vi "Configure Thermistor [THM].vi"(8 "error in (no error)":errorcluster, 10 "resistance (0.0 ohms)":dbl format="%^.2e", 11 "CS++DMM in":refnum<class "CS++DMM.lvclass">) -> (0 "error out":errorcluster, 3 "CS++DMM out":refnum<class "CS++DMM.lvclass">)   [LabVIEW 2013, in "CS++DMM.lvlib" / "CS++DMM.lvclass"]
doc: "This VI configures the resistance for a thermistor temperature measurement device.\n\nThis VI affects the behavior of the instrument only when the IviDmm>Temperature Measurements>Transducer Type [TMP] property is set to IVIDMM_VAL_THERMISTOR.\n\nNote:\n\n(1) This VI is part of the IviDmmThermistor [THM] extension group."
uses:
  CS++DMM.lvclass
  Core/Classes/CS++ProcessVariables/ProcessVariable/PV.lvclass
  Core/Classes/CS++ProcessVariables/ProcessVariable/PV.lvclass/PV.ctl
  CS++DMM.lvclass/CS++DMM.ctl
  Core/Classes/CS++ProcessVariables/PVConnection/PVConnection.lvclass
  Core/Classes/CS++ProcessVariables/ProcessVariable/Write Data.vi
  Core/Classes/CS++ProcessVariables/ProcessVariable/Write Timestamp.vi
  Core/Classes/CS++ProcessVariables/ProcessVariable/Write Quality.vi
  Core/Classes/CS++ProcessVariables/ProcessVariable/Write status.vi
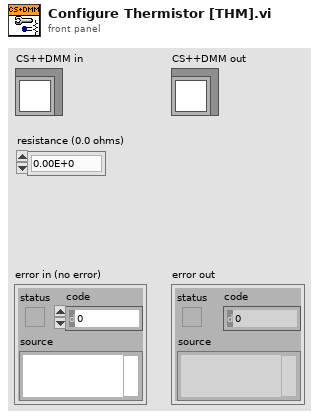
[diagram p1: front panel]
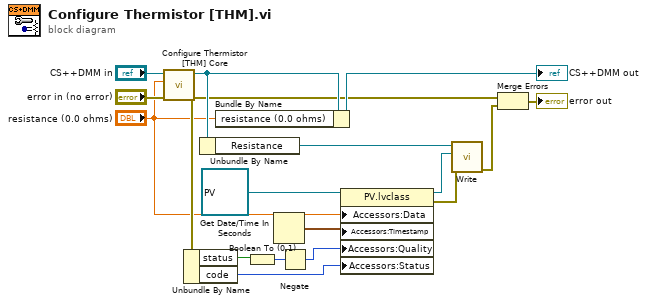
[diagram p0: block diagram]
diagram:
  n1 = call-dynamic "Configure Thermistor [THM] Core.vi"("error in (no error)"="error in (no error)", "resistance (0.0 ohms)"="resistance (0.0 ohms)", "CS++DMM in"="CS++DMM in") -> ("error out"=w4:errorcluster, "CS++DMM out"=w5:refnum<class "CS++DMM.lvclass">)  [unwired: 7 in]
  n2 = Unbundle By Name(w4) -> ("status"=w13:bool, "code"=w10:i32)
  n3 = Unbundle By Name(w5) -> ("Resistance"=w8:refnum<class "PVConnection.lvclass">)
  n4 = Bundle By Name(cluster=w5, "resistance (0.0 ohms)"="resistance (0.0 ohms)") -> (→"CS++DMM out":refnum<class "CS++DMM.lvclass">)
  n5 = Boolean To (0,1)(Boolean=w13) -> (0, 1=w12:i16)
  n6 = Get Date/Time In Seconds() -> (seconds since 1Jan1904=w9:timestamp)
  n7 = Negate(x=w12) -> (-x=w11:i16)
  n8 = property class="PV.lvclass"(reference=refnum<class "PV.lvclass"> refnum ("CS++ProcessVariables.lvlib:PV.lvclass"), "Accessors:Data"="resistance (0.0 ohms)", "Accessors:Timestamp"=w9, "Accessors:Quality"=w11, "Accessors:Status"=w10) -> (reference out=w7:refnum<class "PV.lvclass">, error out=w6:errorcluster)  [unwired: 1 in]
  n9 = call-dynamic "Write.vi"("error in (no error)"=w6, "PV"=w7, "PVConnection in"=w8) -> ("error out"=w1:errorcluster)  [unwired: 7 in, 1 out]
  n10 = Merge Errors(w4, w1) -> (→"error out":errorcluster)
